vi "isSysTopic.vi"(8 "error in (no error)":errorcluster, 10 "Topic":string, 11 "MQTTclient in":refnum<class "MQTTclient.lvclass">) -> (0 "error out":errorcluster, 2 "isSys?":bool, 3 "MQTTclient out":refnum<class "MQTTclient.lvclass">)   [LabVIEW 2017, in "MQTTclient.lvclass"]
uses:
  MQTTclient.lvclass
  MQTTclient.lvclass/MQTTclient.ctl
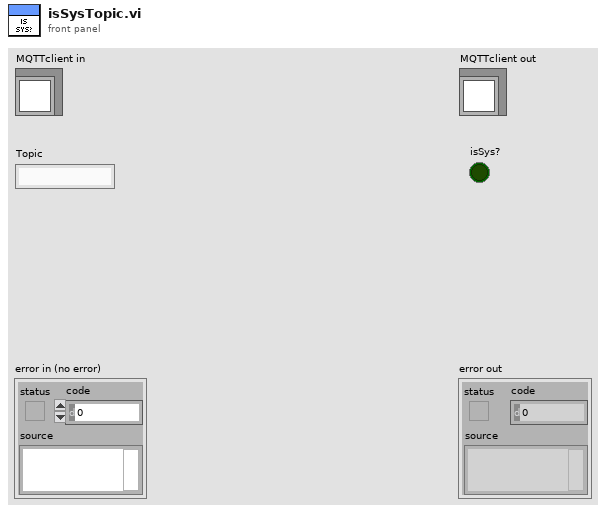
[diagram p1: front panel]
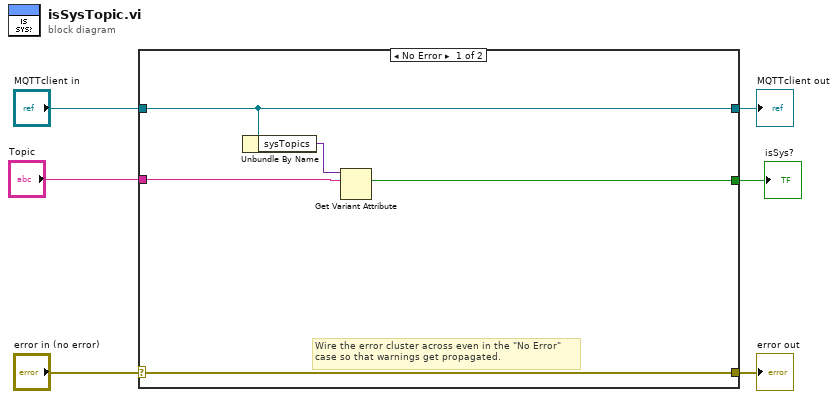
[diagram p0: block diagram]
diagram:
  n1 = case shown="No Error" "error in (no error)" {
    selector: "error in (no error)" -> [w11 w13]
    tunnel: [w11 w13] -> w5
    tunnel: [w10 w12] -> w3
    tunnel: "MQTTclient in" -> [w10 w12]
    tunnel: "Topic" -> [w8 _]
    tunnel: [w7 _] -> w1
    frame No Error {
      # "Wire the error cluster across even in the \"No Error\"\ncase so that warnings get propagated."
      n2 = Unbundle By Name(w10) -> ("sysTopics"=w9:variant)
      n3 = Get Variant Attribute(Variant=w9, name=w8) -> (found=w7:bool)  [unwired: 2 in, 3 out]
    }
    frame Error {
    }
  }
  "error out" <- w5
  "MQTTclient out" <- w3
  "isSys?" <- w1
